vi "Full PC Build.vi"   [LabVIEW 2020]
uses:
  lv-builder/Builder Tools/Builder/Builder.lvclass
  lv-builder/Builder Tools/Simple Build GUI/Simple Build GUI.lvclass
panel:
  # "Full PC Build"
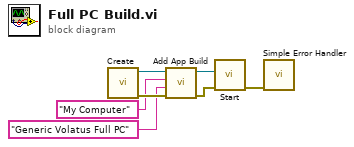
[diagram p0: block diagram]
diagram:
  n1 = call "Create.vi"() -> ("error out"=w7:errorcluster, "Builder out"=w6:refnum<class "Builder.lvclass">)  [unwired: 10 in]
  n2 = call "Add App Build.vi"("error in (no error)"=w7, "Build Spec"="Generic Volatus Full PC" ("Target"), "Target"="My Computer", "Builder in"=w6) -> ("error out"=w4:errorcluster, "Builder out"=w3:refnum<class "Builder.lvclass">)  [unwired: 6 in]
  n3 = call "Start.vi"("error in (no error)"=w4, "Builder"=w3) -> ("error out"=w1:errorcluster)  [unwired: 8 in, 1 out]
  n4 = call <vilib>:"Simple Error Handler.vi"("error in (no error)"=w1) -> ()  [unwired: 4 in, 5 out]
